vi "Set 5-bar Parameters.vi"(8 "error in (no error)":errorcluster, 10 "5-bar Parameters":T1, 11 "Finger in":refnum<class "Finger.lvclass">) -> (0 "error out":errorcluster, 3 "Finger out":refnum<class "Finger.lvclass">)   [LabVIEW 2013, in "Finger.lvclass"]
uses:
  Finger.lvclass
  controls/5-bar Parameters.ctl
  Finger.lvclass/Finger.ctl
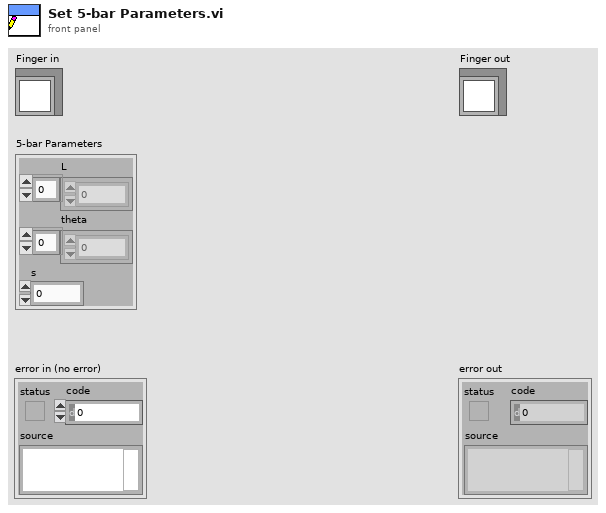
[diagram p1: front panel]
types:
  T1 = typedef "5-bar Parameters.ctl" = cluster{"L":dbl[], "theta":dbl[], "s":dbl}
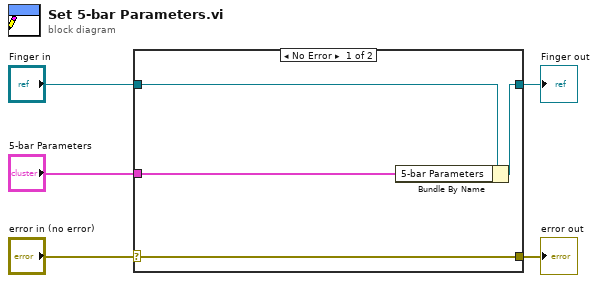
[diagram p0: block diagram]
diagram:
  n1 = case shown="No Error" "error in (no error)" {
    selector: "error in (no error)" -> [w9 w10]
    tunnel: [w9 w10] -> w4
    tunnel: [w7 w11] -> w2
    tunnel: "Finger in" -> [w8 w11]
    tunnel: "5-bar Parameters" -> [w6 _]
    frame No Error {
      n2 = Bundle By Name(cluster=w8, "5-bar Parameters"=w6) -> (w7:refnum<class "Finger.lvclass">)
    }
    frame Error {
    }
  }
  "error out" <- w4
  "Finger out" <- w2
